vi "Knife_Edge_Scan_Parameters_MR.vi"(0 "VISA Ressource in":refnum<visa-resource-name>="COM17", 1 "Axis":u16(ring) items=["Detector", "X-Rays", "Vertical", "In-Plain", "Vertical (with tilt)"], 5 "Scan Range (mum)":dbl=100.0, 7 "Nr. of Steps":u32=10, 9 "Z tilt (angle)":dbl, 11 "error in (no error)":errorcluster, 12 "Echo Mode":i32) -> (2 "V_max 1/3 and 2":i32[](array[numeric]), 3 "(negative) [scan range in steps + one extra step]":string, 4 "VISA ressource out":refnum<visa-resource-name>, 6 "micron steps":dbl[](array[numeric]), 8 "single steps 1":i32[](array[numeric]), 10 "single steps 2":i32[](array[numeric]), 13 "(negative) [scan range in steps]":string, 14 "move time (ms)":u32, 15 "error out":errorcluster={"status"=FALSE, "code"=1073676294, "source"="VISA Read in write_read.vi"})   [LabVIEW 2015]
uses:
  ConversionAndInformation/Unit_Control.ctl
  MCode_LV_86/Set Parameter.ctl
panel:
  out "angle":dbl
  out "delta angle":dbl
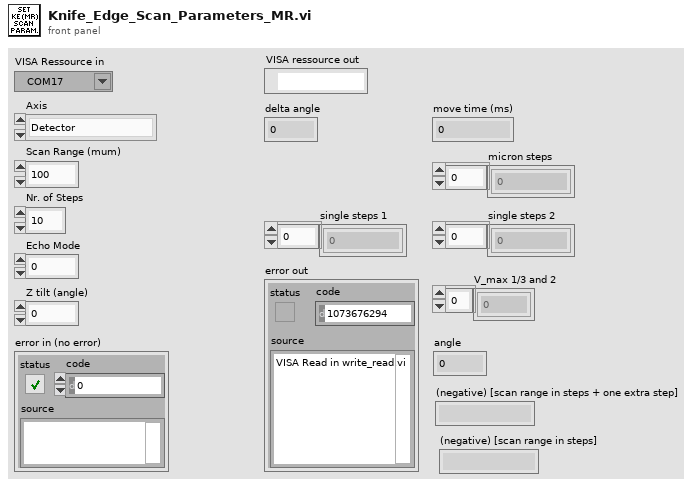
[diagram p1: front panel]
types:
  T1 = typedef "Unit_Control.ctl" = enum16{"Angle (Degrees)", "Rad", "Angle [TMC]", "Microsteps [TMC]", "Inches", "Nanometer", "Meter", "Centimeter", "Millimeter", "Micron"}
  T2 = typedef "Set Parameter.ctl" = enum16{"Acceleration (A)", "Baud Rate (BD)", "Counter 1 (C1)", "Counter 2 (C2)", "Control C Software Reset (CE)", "Check Sum Enable (CK)", "Clock Mode (CM)", "Clock Mode Ratio (CR)", "Clock Mode Out Step Width (CW)", "Deceleration (D)", "Digital Filtering, Input 1 (D1)", "Digital Filtering, Input 2 (D2)", "Digital Filtering, Input 3 (D3)", "Digital Filtering, Input 4 (D4)", "Digital Filtering, Input 5 (D5)", "Digital Filtering, Input 9 (D9)", "Digital Filtering, Input 10 (D10)", "Digital Filtering, Input 11 (D11)", "Digital Filtering, Input 12 (D12)", "Deadband (DB)", "Decrement Variable (DC)", "Enable/Disable Drive (DE)", "Device Name (DN)", "End Program Execution (E)", "Encoder Function Enable (EE)", "Error Flag (EF)", "Encoder Lines (EL)", "Echo Mode (EM)", "Error Value (ER)", "Escape (ES)", "Execute Program at Address (EX)", "Firmware Version (VR)", "Hold (H)", "Hold Current (HC)", "Hold Current Delay Time (HI)", "Home to Encoder Index (HM)", "Home to Home Switch (HT)", "Increment Variable (IC)", "Initialize Parameters to NVM (IP)", "Input into Variable (IV)", "Jog Enable (JE)", "Limit Stop Mode (LM)", "Move Absolute (MA)", "Move Relative (MR)", "MicroStepping Select (MS)", "Motor Settling Delay Time (MT)", "Moving [Flag] (MV)", "Output 1 (O1)", "Output 2 (O2)", "Output 3 (O3)", "Output 4 (O4)", "Output 9 (O9)", "Output 10 (O10)", "Output 11 (O11)", "Output 12 (O12)", "Output High Byte (9-12) (OH)", "Output Low Byte (1-4) (OL)", "Output Total (1-4 and 9-12) (OT)", "Position (P)", "Position Maintenance (PM)", "Party Mode (PY)", "Register 1 (R1)", "Register 2 (R2)", "Register 3 (R3)", "Register 4 (R4)", "Reset Error(\\03)", "Run Current (RC)", "Stall Factor (SF)", "Slew (SL)", "Stall Mode Set (SM)", "Upgrade Firmware (UG)", "Velocity Initial (VI)", "Velocity Maximum (VM)"}
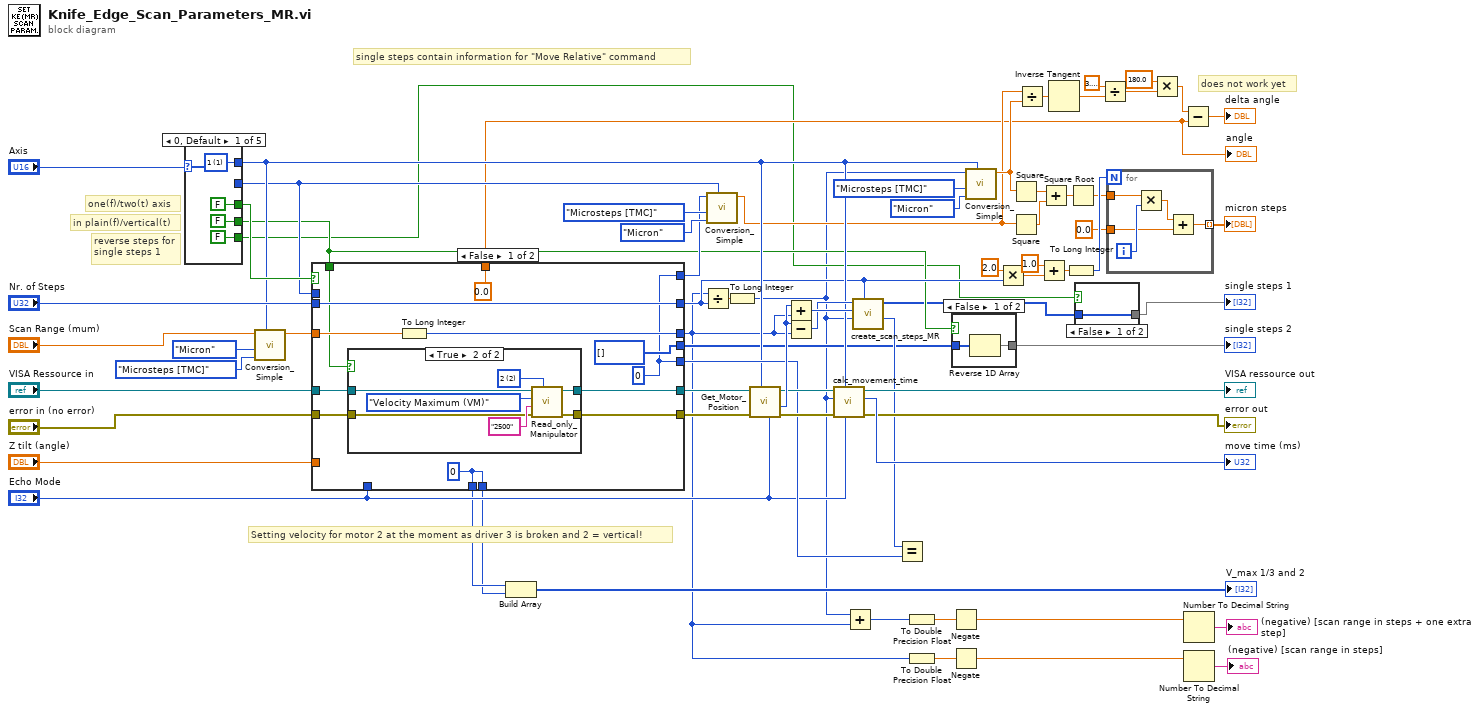
[diagram p0: block diagram]
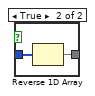
[diagram p2: hidden frame]
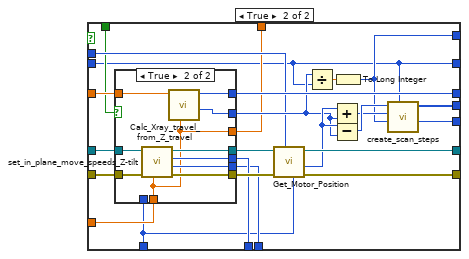
[diagram p5: hidden frame]
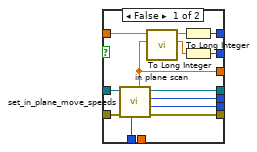
[diagram p6: hidden frame]
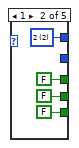
[diagram p7: hidden frame]
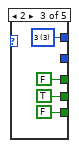
[diagram p8: hidden frame]
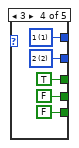
[diagram p9: hidden frame]
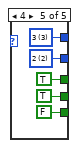
[diagram p10: hidden frame]
diagram:
  # "Setting velocity for motor 2 at the moment as driver 3 is broken and 2 = vertical!"
  # "single steps contain information for \"Move Relative\" command"
  # "reverse steps for\nsingle steps 1"
  # "does not work yet"
  # "in plain(f)/vertical(t)"
  # "one(f)/two(t) axis"
  n1 = case shown="0, Default" "Axis" {
    tunnel: [w75 w79 w83 w88 w93] -> w45
    tunnel: [_ _ _ w87 w92] -> w42
    tunnel: [FALSE FALSE FALSE TRUE TRUE] -> w52
    tunnel: [FALSE FALSE TRUE FALSE TRUE] -> w14
    tunnel: [FALSE FALSE FALSE FALSE FALSE] -> w10
    frame 0, Default {
      w75 = u16 1 items=["none", "1", "2", "3", "4", "all"] ("Motor")
    }
    frame 1 {
      w79 = u16 2 items=["none", "1", "2", "3", "4", "all"] ("Motor")
    }
    frame 2 {
      w83 = u16 3 items=["none", "1", "2", "3", "4", "all"] ("Motor")
    }
    frame 3 {
      w87 = u16 2 items=["none", "1", "2", "3", "4", "all"] ("Motor")
      w88 = u16 1 items=["none", "1", "2", "3", "4", "all"] ("Motor")
    }
    frame 4 {
      w92 = u16 2 items=["none", "1", "2", "3", "4", "all"] ("Motor")
      w93 = u16 3 items=["none", "1", "2", "3", "4", "all"] ("Motor")
    }
  }
  n2 = call "Conversion_Simple.vi"("Motor"=w45, "Output Unit"=Unit_Control."Microsteps [TMC]", "Input Unit"=Unit_Control."Micron", "Input"="Scan Range (mum)") -> ("Output"=w63:dbl)  [unwired: 6 in, 1 out]
  n3 = case shown="False" w52 {
    tunnel: w63 -> [w104 w138]
    tunnel: [w97 w137] -> w62
    tunnel: [w95 w136] -> w61
    tunnel: [w105 w133] -> w25
    tunnel: [w105 w132] -> w24
    tunnel: [i32[] [] ("single steps") w128] -> w16
    tunnel: [w103 w126] -> w2
    tunnel: [w100 w124] -> w59
    tunnel: w42 -> [_ w123]
    tunnel: "Nr. of Steps" -> [w101 w115]
    tunnel: "VISA Ressource in" -> [w98 w122]
    tunnel: "error in (no error)" -> [w96 w121]
    tunnel: "Echo Mode" -> [_ w118]
    tunnel: w14 -> [w94 w120]
    tunnel: "Z tilt (angle)" -> [_ w119]
    tunnel: [w101 w115] -> w17
    tunnel: [w100 w117] -> w41
    tunnel: [0.0 w116] -> w13
    frame False {
      w100 = 0 ("array length")
      w105 = 0 ("V_max Motor 3")
      n4 = case shown="True" w94 {
        tunnel: w98 -> [w107 w112]
        tunnel: [w107 w111] -> w97
        tunnel: w96 -> [w106 w110]
        tunnel: [w106 w109] -> w95
        frame False {
        }
        frame True {
          w113 = u16 2 items=["none", "1", "2", "3", "4", "all"] ("Motor")
          n5 = call "Read_only_Manipulator.vi"("Motor"=w113, "error in (no error)"=w110, "Value"="2500", "Command"=Set_Parameter."Velocity Maximum (VM)", "VISA resource name"=w112) -> ("error out"=w109:errorcluster, "VISA ressource out"=w111:refnum<visa-resource-name>)  [unwired: 3 in, 2 out]
        }
      }
      n6 = To Long Integer(number=w104) -> (32bit integer=w103:i32)
    }
    frame True {
      n7 = case shown="True" w120 {
        tunnel: w138 -> [w151 w155]
        tunnel: [w150 w159] -> w135
        tunnel: [w149 w158] -> w134
        tunnel: [w148 w157] -> w133
        tunnel: [w147 w156] -> w132
        tunnel: [w144 w154] -> w126
        tunnel: [w143 w153] -> w125
        tunnel: w122 -> [w142 w161]
        tunnel: w121 -> [w141 w160]
        tunnel: w118 -> [w140 _]
        tunnel: w119 -> [_ w152]
        tunnel: [w139 w152] -> w116
        frame False {
          n8 = call "set_in_plane_move_speeds.vi"("Echo Mode"=w140, "error in (no error)"=w141, "VISA resource name"=w142) -> ("error out"=w149:errorcluster, "V_max Motor 2"=w147:i32, "V_max Motor 1"=w148:i32, "VISA ressource out"=w150:refnum<visa-resource-name>, "Angle Sample Holder"=w139:dbl)  [unwired: 4 in]
          n9 = call "in plane scan.vi"("angle (degrees)"=w139, "v total"=w151) -> ("v_y"=w146:dbl, "v_x"=w145:dbl)  [unwired: 4 in, 4 out]
          n10 = To Long Integer(number=w145) -> (32bit integer=w144:i32)
          n11 = To Long Integer(number=w146) -> (32bit integer=w143:i32)
        }
        frame True {
          n12 = call "set_in_plane_move_speeds_Z-tilt.vi"("Z tilt (angle)"=w152, "error in (no error)"=w160, "VISA resource name"=w161) -> ("error out"=w158:errorcluster, "V_max Motor 2"=w156:i32, "V_max Motor 3"=w157:i32, "VISA ressource out"=w159:refnum<visa-resource-name>)  [unwired: 5 in]
          n13 = call "Calc_Xray_travel_from_Z_travel.vi"("Z tilt (degrees)"=w152, "Z travel (steps)"=w155) -> ("X-ray travel (steps)"=w153:i32, "Z travel (steps)"=w154:i32)  [unwired: 8 in]
        }
      }
      n14 = call "Get_Motor_Position.vi"("Echo Mode (2)"=w118, "Motor In"=w123, "error in (no error)"=w134, "VISA resource name"=w135) -> ("error out"=w136:errorcluster, "Position (Steps)"=w129:i32, "VISA ressource out"=w137:refnum<visa-resource-name>)  [unwired: 4 in, 1 out]
      n15 = Divide(x=w125, y=w115) -> (x/y=w127:dbl)
      n16 = Add(x=w129, y=w125) -> (x+y=w130:i32)
      n17 = Subtract(x=w129, y=w125) -> (x-y=w131:i32)
      n18 = To Long Integer(number=w127) -> (32bit integer=w117:i32)
      n19 = call "create_scan_steps.vi"("number of steps"=w115, "step"=w117, "stop"=w130, "start"=w131) -> ("array length"=w124:i32, "single steps"=w128:i32[])  [unwired: 6 in]
    }
  }
  "angle" <- w13
  n20 = Build Array(w25, w24) -> (→"V_max 1/3 and 2":i32[])
  n21 = Divide(x=w2, y=w17) -> (x/y=w60:dbl)
  n22 = call "Conversion_Simple.vi"("Motor"=w42, "Output Unit"=Unit_Control."Micron", "Input Unit"=Unit_Control."Microsteps [TMC]", "Input"=w41) -> ("Output"=w26:dbl)  [unwired: 6 in, 1 out]
  n23 = To Long Integer(number=w60) -> (32bit integer=w6:i32)
  n24 = call "Get_Motor_Position.vi"("Echo Mode (2)"="Echo Mode", "Motor In"=w45, "error in (no error)"=w61, "VISA resource name"=w62) -> ("error out"=w66:errorcluster, "Position (Steps)"=w67:i32, "VISA ressource out"=w65:refnum<visa-resource-name>)  [unwired: 4 in, 1 out]
  n25 = Add(x=w67, y=w2) -> (x+y=w71:i32)
  n26 = Subtract(x=w67, y=w2) -> (x-y=w70:i32)
  n27 = call "calc_movement_time.vi"("Echo Mode"="Echo Mode", "Motor"=w45, "error in (no error)"=w66, "steps"=w6, "VISA ressource in"=w65) -> ("error out"=→"error out":errorcluster, "move time (ms)"=→"move time (ms)":u32, "VISA ressource out"=→"VISA ressource out":refnum<visa-resource-name>)  [unwired: 3 in, 1 out]
  n28 = Add(x=w6, y=w2) -> (x+y=w5:i32)
  n29 = call "create_scan_steps_MR.vi"("number of steps"=w17, "step"=w6, "stop"=w71, "start"=w70) -> ("array length"=w48:i32, "single steps"=w12:i32[])  [unwired: 6 in]
  n30 = Equal?(x=w48, y=w59) -> ()  [unwired: 1 out]
  n31 = To Double Precision Float(number=w5) -> (double precision float=w8:dbl)
  n32 = To Double Precision Float(number=w2) -> (double precision float=w3:dbl)
  n33 = Negate(x=w8) -> (-x=w7:dbl)
  n34 = Negate(x=w3) -> (-x=w4:dbl)
  n35 = case shown="False" w14 {
    tunnel: w16 -> [w163 w164]
    tunnel: [w162 w164] -> w15
    frame False {
      n36 = Reverse 1D Array(array=w163) -> (reversed array=w162:i32[])
    }
    frame True {
    }
  }
  "single steps 2" <- w15
  n37 = call "Conversion_Simple.vi"("Motor"=w45, "Output Unit"=Unit_Control."Micron", "Input Unit"=Unit_Control."Microsteps [TMC]", "Input"=w6) -> ("Output"=w27:dbl)  [unwired: 6 in, 1 out]
  n38 = Multiply(x=2.0, y=w17) -> (x*y=w35:dbl)
  n39 = Square(x=w27) -> (x^2=w40:dbl)
  n40 = Square(x=w26) -> (x^2=w39:dbl)
  n41 = Divide(x=w26, y=w27) -> (x/y=w28:dbl)
  n42 = Add(x=1.0, y=w35) -> (x+y=w33:dbl)
  n43 = Add(x=w40, y=w39) -> (x+y=w38:dbl)
  n44 = Inverse Tangent(1:w28) -> (0:w21:dbl)
  n45 = To Long Integer(number=w33) -> (32bit integer=w32:i32)
  n46 = Square Root(x=w38) -> (sqrt(x)=w30:dbl)
  n47 = case shown="False" w10 {
    tunnel: w12 -> [w165 w167]
    tunnel: [w165 w166] -> w11
    frame False {
    }
    frame True {
      n48 = Reverse 1D Array(array=w167) -> (reversed array=w166:i32[])
    }
  }
  "single steps 1" <- w11
  n49 = Divide(x=3.141592653589793, y=w21) -> (x/y=w20:dbl)
  n50 = for {
    N: w32 -> [_]
    tunnel: 0.0 -> [w170]
    tunnel: w30 -> [w172]
    tunnel: [w168] -> w29 mode=indexing
    i -> [w171]
    n51 = Multiply(x=w172, y=w171) -> (x*y=w169:dbl)
    n52 = Add(x=w169, y=w170) -> (x+y=w168:dbl)
  }
  "micron steps" <- w29
  n53 = Multiply(x=180.0 ("y"), y=w20) -> (x*y=w18:dbl)
  n54 = Subtract(x=w18, y=w13) -> (x-y=→"delta angle":dbl)
  n55 = Number To Decimal String(number=w7) -> (decimal integer string=→"(negative) [scan range in steps + one extra step]":string)  [unwired: 1 in]
  n56 = Number To Decimal String(number=w4) -> (decimal integer string=→"(negative) [scan range in steps]":string)  [unwired: 1 in]
